vi "ComSerialArduino.vi"() -> ()   [LabVIEW 2024]
uses:
  Lib/cluster_DataArduino.ctl
panel:
  out "DataRX":string
  in  "parametre":string
  in  "fonction":string
  in  "Test envoi":bool
  in  "endChar":string=";"
  in  "syncChar":string="@"
  in  "stop":bool
  in  "port COM arduino":refnum<visa-resource-name>
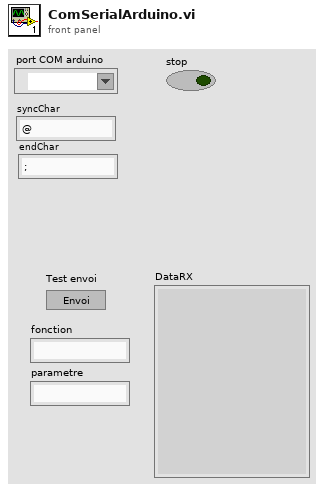
[diagram p1: front panel]
types:
  T1 = typedef "cluster_DataArduino.ctl" = cluster{"adresse":i32, "fonction":string, "parametre":string}
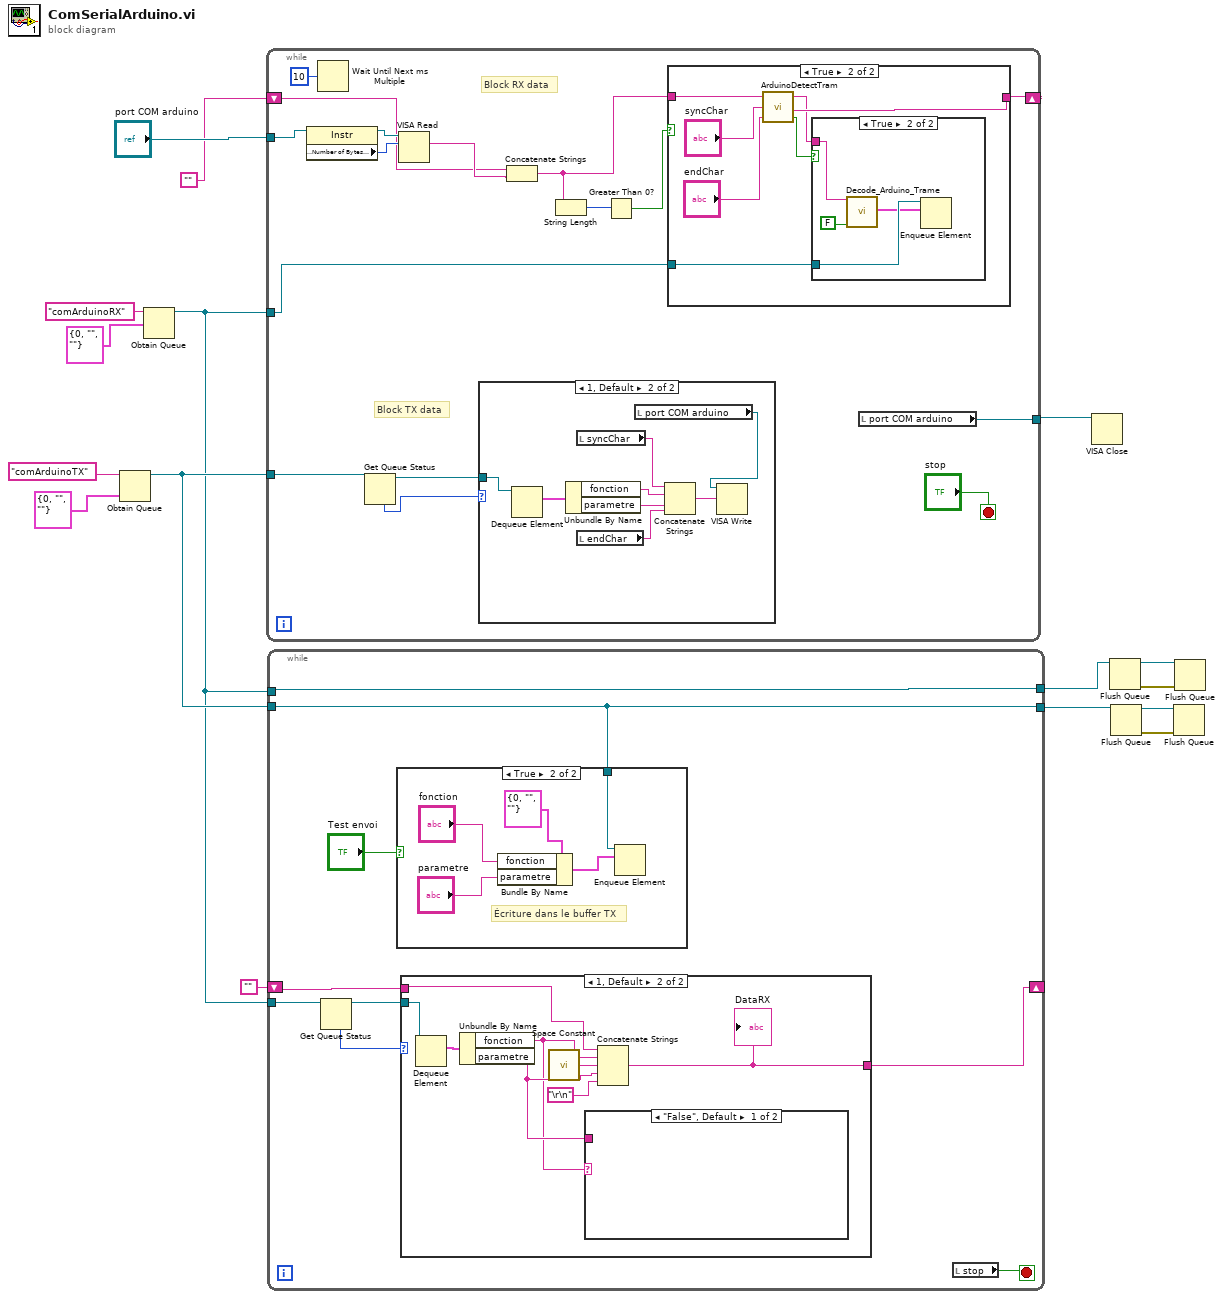
[diagram p0: block diagram]
diagram:
  n1 = Obtain Queue(name (unnamed)="comArduinoTX", element data type=T1 {"adresse"=0, "fonction"="", "parametre"=""} ("clusterDataArduino")) -> (queue out=w9:refnum<queue>)  [unwired: 3 in, 2 out]
  n2 = Obtain Queue(name (unnamed)="comArduinoRX", element data type=T1 {"adresse"=0, "fonction"="", "parametre"=""} ("clusterDataArduino")) -> (queue out=w2:refnum<queue>)  [unwired: 3 in, 2 out]
  n3 = while {
    tunnel: "port COM arduino" -> [w30]
    shift-right: [w22] -> _
    shift-left: "" -> [w27]
    tunnel: w2 -> [w21]
    tunnel: w9 -> [w20]
    tunnel: [w17] -> w10
    stop <- "stop" stop-if-true
    # "Block RX data"
    # "Block TX data"
    n4 = property class="Instr"(reference=w30) -> (reference out=w31:refnum<visa-resource-name>, "Serial Settings:Number of Bytes at Serial Port"=w32:u32)  [unwired: 1 in, 1 out]
    n5 = Wait Until Next ms Multiple(millisecond multiple=u32 10) -> ()  [unwired: 1 out]
    n6 = Get Queue Status(queue=w20) -> (queue out=w18:refnum<queue>, # elements in queue=w19:i32)  [unwired: 2 in, 6 out]
    n7 = VISA Read(VISA resource name=w31, byte count=w32) -> (read buffer=w28:string)  [unwired: 1 in, 3 out]
    n8 = case shown="1, Default" w19 {
      tunnel: w18 -> [_ w40]
      frame 0 {
      }
      frame 1, Default {
        n9 = Dequeue Element(queue=w40) -> (element=w39:T1)  [unwired: 2 in, 3 out]
        n10 = Unbundle By Name(w39) -> ("fonction"=w37:string, "parametre"=w36:string)
        n11 = local read "syncChar"() -> (w38:string)
        n12 = local read "endChar"() -> (w35:string)
        n13 = local read "port COM arduino"() -> (w33:refnum<visa-resource-name>)
        n14 = Concatenate Strings(w38, w37, w36, w35) -> (w34:string)
        n15 = VISA Write(VISA resource name=w33, write buffer=w34) -> ()  [unwired: 1 in, 3 out]
      }
    }
    n16 = Concatenate Strings(w27, w28) -> (w23:string)
    n17 = String Length(string=w23) -> (length=w25:i32)
    n18 = Greater Than 0?(x=w25) -> (x > 0?=w24:bool)
    n19 = case shown="True" w24 {
      tunnel: w23 -> [w41 w48]
      tunnel: [w41 w45] -> w22
      tunnel: w21 -> [_ w42]
      frame False {
      }
      frame True {
        n20 = call "ArduinoDetectTram.vi"("endChar"="endChar", "syncChar"="syncChar", "bufferIN"=w48) -> ("dataDetected"=w44:bool, "bufferOUT"=w45:string, "data"=w43:string)
        n21 = case shown="True" w44 {
          tunnel: w43 -> [_ w49]
          tunnel: w42 -> [_ w52]
          frame False {
          }
          frame True {
            n22 = call "Decode_Arduino_Trame.vi"("arduinoData"=w49, "adressable?"=FALSE) -> ("dataOut"=w50:T1)  [unwired: 10 in, 3 out]
            n23 = Enqueue Element(queue=w52, element=w50) -> ()  [unwired: 2 in, 3 out]
          }
        }
      }
    }
    n24 = local read "port COM arduino"() -> (w17:refnum<visa-resource-name>)
  }
  n25 = while {
    tunnel: w2 -> [w61]
    tunnel: [w61] -> w8
    tunnel: w9 -> [w56]
    tunnel: [w56] -> w7
    tunnel: w2 -> [w60]
    shift-right: [w53] -> _
    shift-left: "" -> [w54]
    stop <- w55 stop-if-true
    n26 = Get Queue Status(queue=w60) -> (queue out=w58:refnum<queue>, # elements in queue=w59:i32)  [unwired: 2 in, 6 out]
    n27 = case shown="True" "Test envoi" {
      tunnel: w56 -> [_ w75]
      frame False {
      }
      frame True {
        # "Écriture dans le buffer TX"
        n28 = Bundle By Name(cluster=T1 {"adresse"=0, "fonction"="", "parametre"=""} ("clusterDataArduino"), "fonction"="fonction", "parametre"="parametre") -> (w74:T1)
        n29 = Enqueue Element(queue=w75, element=w74) -> ()  [unwired: 2 in, 3 out]
      }
    }
    n30 = case shown="1, Default" w59 {
      tunnel: w58 -> [_ w70]
      tunnel: w54 -> [w62 w68]
      tunnel: [w62 w65] -> w53
      frame 0 {
      }
      frame 1, Default {
        n31 = Dequeue Element(queue=w70) -> (element=w69:T1)  [unwired: 2 in, 3 out]
        n32 = Unbundle By Name(w69) -> ("fonction"=w63:string, "parametre"=w64:string)
        n33 = call <vilib>:"Space Constant.vi"() -> ("String"=w67:string)
        n34 = case shown="\"False\", Default" w63 {
          tunnel: w64 -> [_ _]
          frame "False", Default {
          }
          frame "True" {
          }
        }
        n35 = Concatenate Strings(w68, w63, w67, w64, "\r\n") -> (w65:string)
        "DataRX" <- w65
      }
    }
    n36 = local read "stop"() -> (w55:bool)
  }
  n37 = VISA Close(VISA resource name=w10) -> ()  [unwired: 1 in, 1 out]
  n38 = Flush Queue(queue=w8) -> (queue out=w6:refnum<queue>, error out=w5:errorcluster)  [unwired: 1 in, 1 out]
  n39 = Flush Queue(queue=w7) -> (queue out=w4:refnum<queue>, error out=w3:errorcluster)  [unwired: 1 in, 1 out]
  n40 = Flush Queue(queue=w4, error in (no error)=w3) -> ()  [unwired: 3 out]
  n41 = Flush Queue(queue=w6, error in (no error)=w5) -> ()  [unwired: 3 out]
